vi "MoveWindow(SubVI).vi"(8 "error in (no error)":errorcluster, 11 "hWnd":u32) -> (0 "error out":errorcluster)   [LabVIEW 2010]
uses:
  user32.dll
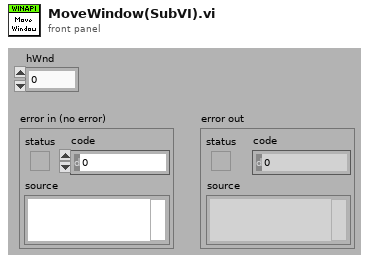
[diagram p1: front panel]
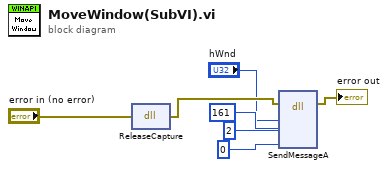
[diagram p0: block diagram]
diagram:
  n1 = dll-call lib="user32.dll" fn="ReleaseCapture"(error in="error in (no error)") -> (error out=w7:errorcluster)  [unwired: 3 in, 1 out]
  n2 = dll-call lib="user32.dll" fn="SendMessageA"(error in=w7, "hWnd"="hWnd", "Msg"=161, "wParam"=2, "lParam"=0) -> (error out=→"error out":errorcluster)  [unwired: 7 in, 1 out]
